vi "期末11 (1).vi"() -> ()   [LabVIEW 2014]
uses:
  <vilib>/vision/NI_Vision_Development_Module.lvlib
panel:
  in  "計數器":dbl
  out "座標和":dbl
  out "output array":dbl[](array[numeric])
  out "x/y":dbl
  out "Image Out 2":T1(plugin-control)
  out "ROI":T2
  in  "紀錄中點座標和":bool
  out "填入飽和磁場分量尖點座標和 2":dbl
  in  "3. Number of Erosion":i32=10
  out "Image Out":T1(plugin-control)
  in  "紀錄電流":dbl[](array[numeric])
  in  "Tab Control 2":enum32{"座標", "座標和", "作圖"}(tab)
  out "瞬間尖點座標":dbl[][](array[numeric])
  out "尖點座標和":dbl[](array[numeric])
  out "相減結果":dbl[](array[numeric])
  out "分量-電流":cluster{"紀錄電流":dbl[], dbl[]}(graph)
  in  "紀錄":bool
  in  "結束實驗":bool
  in  "1. 範圍選擇":T3={"色相（H）"={0, 255}, "飽和度（S）"={0, 255}, "亮度（L）"={0, 255}} {"亮度（L）" scale=0.0..255.0; "飽和度（S）" scale=0.0..255.0; "色相（H）" scale=0.0..255.0}
  out "Number of Particles":i32
  out "output cluster":cluster{"X":dbl, "Y":dbl}
  in  "Tab Control":T4(tab)
  out "1. 顏色選取":T1(plugin-control)
  out "2. 填補空隙":T1(plugin-control)
  out "3. 移除雜點":T1(plugin-control)
  out "4. 形狀修正":T1(plugin-control)
  out "5. 選取結果":T1(plugin-control)
  out "Particle Measurements":dbl[][](array[numeric])
  out "Error Out":errorcluster
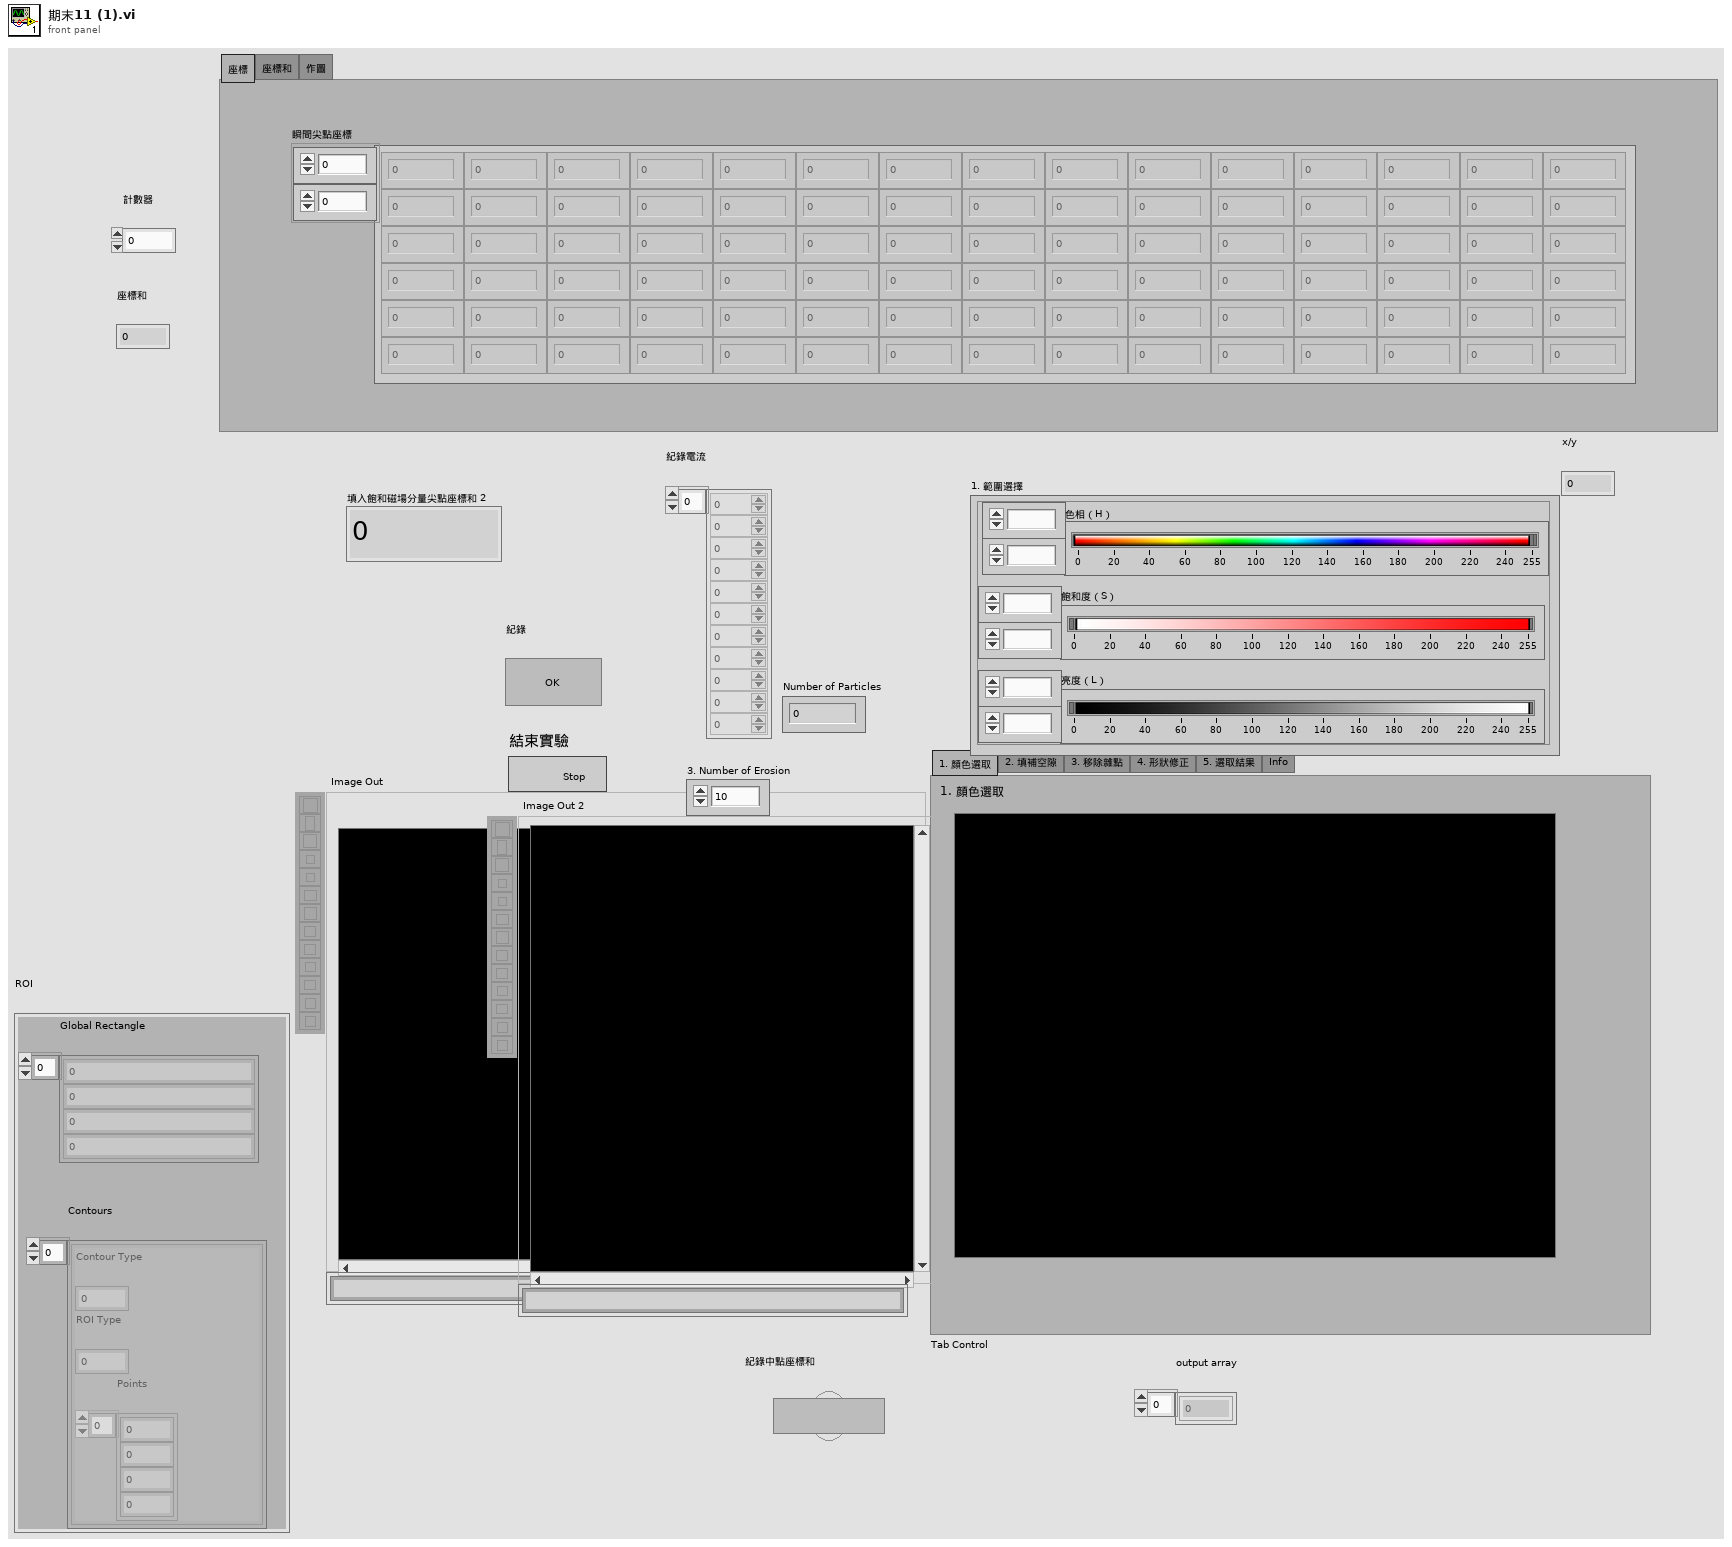
[diagram p1: front panel]
types:
  T1 = typedef "IMAQ Image.ctl" = refnum<image>
  T2 = cluster{"Global Rectangle":i32[], "Contours":cluster{"Contour Type":u32, "ROI Type":u32, "Points":i32[]}[]}
  T3 = cluster{"色相（H）":cluster{u8, u8}, "飽和度（S）":cluster{u8, u8}, "亮度（L）":cluster{u8, u8}}
  T4 = enum32{"1. 顏色選取", "2. 填補空隙", "3. 移除雜點", "4. 形狀修正", "5. 選取結果", "Info"}
  T5 = typedef "Image Type" = u32
  T6 = cluster{"Numeric":dbl, "Numeric":dbl, "Numeric":dbl, "Numeric":dbl}
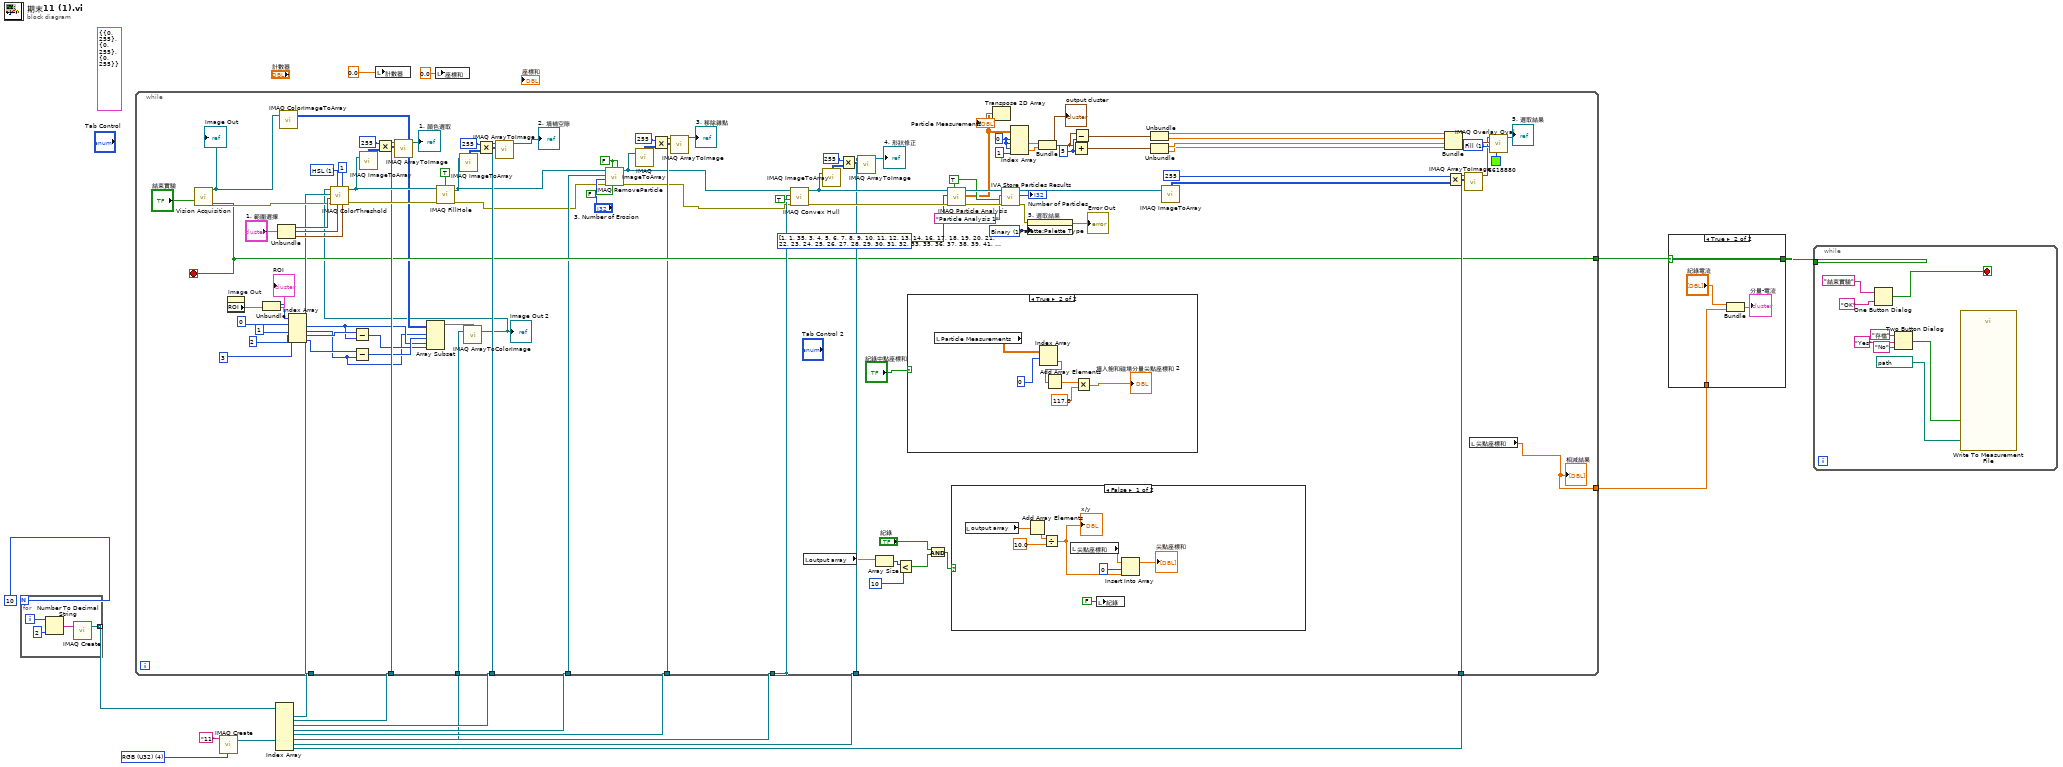
[diagram p0: block diagram]
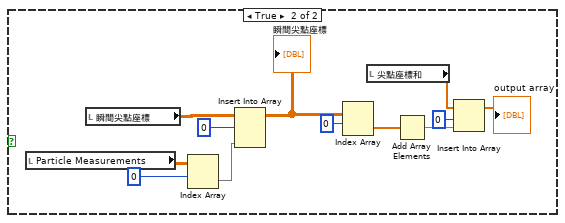
[diagram p3: hidden frame]
diagram:
  w5 = T5 4 items=["Grayscale (U8)", "Grayscale (I16)", "Grayscale (SGL)", "Complex (CSG)", "RGB (U32)", "HSL (U32)", "RGB (U64)", "Grayscale (U16)"] ("Image Type")
  (unwired) T3 {"色相（H）"={0, 255}, "飽和度（S）"={0, 255}, "亮度（L）"={0, 255}} ("範圍選擇")
  n1 = for {
    N: 10 -> [_]
    tunnel: [w19] -> w18 mode=indexing
    i -> [w21]
    n2 = Number To Decimal String(number=w21, width (-)=2) -> (decimal integer string=w20:string)
    n3 = call "IMAQ Create"("Image Name"=w20) -> ("New Image"=w19:T1)  [unwired: 4 in, 1 out]
  }
  n4 = call "IMAQ Create"("Image Name"="11", "Image Type"=w5) -> ("New Image"=w6:T1)  [unwired: 3 in, 1 out]
  n5 = Index Array(array=w18) -> (element #1=w17:T1, element #2=w16:T1, element #3=w15:T1, element #4=w8:T1, element #5=w7:T1, element #6=w13:T1, element #7=w12:T1, element #8=w11:T1)  [unwired: 8 in]
  n6 = while {
    tunnel: w15 -> [w95]
    tunnel: w13 -> [w106]
    tunnel: [w106] -> _
    tunnel: w16 -> [w100]
    tunnel: w17 -> [w94]
    tunnel: w12 -> [w88]
    tunnel: w11 -> [w65]
    tunnel: [w61] -> w10
    tunnel: [w47] -> w9
    tunnel: w8 -> [w54]
    tunnel: w7 -> [w53]
    tunnel: w6 -> [w37]
    stop <- w61 stop-if-true
    w58 = FALSE ("Connectivity 4/8 (8)")
    w70 = u32 1 items=["Frame", "Fill"] ("Drawing Mode (Frame)")
    w79 = 5
    w84 = 0
    w108 = u32 1 items=["Grayscale", "Binary", "Gradient", "Rainbow", "Temperature", "User Defined"] ("Palette")
    w113 = i32[] [1, 1, 35, 3, 4, 5, 6, 7, 8, 9, 10, 11, 12, 13, 14, 16, 17, 18, 19, 20, 21, 22, 23, 24, 25, 26, 27, 28, 29, 30, 31, 32, 33, 35, 36, 37, 38, 39, 41, 42, 43, 45, 46, 48, 49, 50, 51, 53, 54, 55, 56, 58, 59, 60, 61, 62, 63, 64, 65, 66, 68, 69, 70, 71, 72, 73, 74, 75, 76, 77, 78, 79, 80, 81, 82, 83, 84, 85, 86, 87, 88] items=["Center of Mass X", "Center of Mass Y", "First Pixel X", "First Pixel Y", "Bounding Rect Left", "Bounding Rect Top", "Bounding Rect Right", "Bounding Rect Bottom", "Max Feret Diameter Start X", "Max Feret Diameter Start Y", "Max Feret Diameter End X", "Max Feret Diameter End Y", "Max Horiz. Segment Length Left", "Max Horiz. Segment Length Right", "Max Horiz. Segment Length Row", "-", "Bounding Rect Width", "Bounding Rect Height", "Bounding Rect Diagonal", "Perimeter", "Convex Hull Perimeter", "Holes' Perimeter", "Max Feret Diameter", "Equivalent Ellipse Major Axis", "Equivalent Ellipse Minor Axis", "Equivalent Ellipse Minor Axis (Feret)", "Equivalent Rect Long Side", "Equivalent Rect Short Side", "Equivalent Rect Diagonal", "Equivalent Rect Short Side (Feret)", "Average Horiz. Segment Length", "Average Vert. Segment Length", "Hydraulic Radius", "Waddel Disk Diameter", "-", "Area", "Holes' Area", "Particle & Holes' Area", "Convex Hull Area", "Image Area", "-", "Number of Holes", "Number of Horiz. Segments", "Number of Vert. Segments", "-", "Orientation", "Max Feret Diameter Orientation", "-", "% Area/Image Area", "% Area/(Particle & Holes' Area)", "Ratio of Equivalent Ellipse Axes", "Ratio of Equivalent Rect Sides", "-", "Elongation Factor", "Compactness Factor", "Heywood Circularity Factor", "Type Factor", "-", "Sum X", "Sum Y", "Sum XX", "Sum XY", "Sum YY", "Sum XXX", "Sum XXY", "Sum XYY", "Sum YYY", "-", "Moment of Inertia XX", "Moment of Inertia XY", "Moment of Inertia YY", "Moment of Inertia XXX", "Moment of Inertia XXY", "Moment of Inertia XYY", "Moment of Inertia YYY", "Norm. Moment of Inertia XX", "Norm. Moment of Inertia XY", "Norm. Moment of Inertia YY", "Norm. Moment of Inertia XXX", "Norm. Moment of Inertia XXY", "Norm. Moment of Inertia XYY", "Norm. Moment of Inertia YYY", "Hu Moment 1", "Hu Moment 2", "Hu Moment 3", "Hu Moment 4", "Hu Moment 5", "Hu Moment 6", "Hu Moment 7"] ("Pixel Measurements")
    w115 = TRUE ("Connectivity 4/8 (8)")
    w124 = u16 1 items=["RGB", "HSL", "HSV", "HSI"] ("Color Mode")
    n7 = call "Vision Acquisition"("Stop (F)"="結束實驗") -> ("Image Out"=w45:T1, "Stopped"=w61:bool, "error out"=w119:errorcluster)  [unwired: 24 in]
    "Image Out" <- w45
    n8 = property on="Image Out" class="ImageControl"() -> ("ROI"=w43:T2)  [unwired: 2 in, 2 out]
    "ROI" <- w43
    n9 = Unbundle(w43) -> ("Global Rectangle"=w42:i32[])  [unwired: 1 out]
    n10 = Unbundle("1. 範圍選擇") -> ("色相（H）"=w123:cluster{u8, u8}, "飽和度（S）"=w122:cluster{u8, u8}, "亮度（L）"=w121:cluster{u8, u8})
    n11 = call "IMAQ ColorImageToArray"("Image"=w45) -> ("Image Pixels (U32)"=w44:u32[][])  [unwired: 3 in, 2 out]
    n12 = Index Array(array=w42, index #1=0 ("index"), index #2=1 ("index"), index #3=2 ("index"), index #4=3 ("index")) -> (element #1=w32:i32, element #2=w30:i32, element #3=w35:i32, element #4=w31:i32)
    n13 = Subtract(x=w35, y=w32) -> (x-y=w33:i32)
    n14 = Subtract(x=w31, y=w30) -> (x-y=w34:i32)
    n15 = Array Subset(array=w44, index (row)=w30, length (row)=w34, index (col)=w32, length (col)=w33) -> (w36:u32[][])
    n16 = call "IMAQ ArrayToColorImage"("Image Pixels (U32)"=w36, "Image"=w37) -> ("Image Out"=w29:T1)  [unwired: 3 in, 1 out]
    "Image Out 2" <- w29
    n17 = call "IMAQ ColorThreshold"("Blue or Luma or Val or Inten Range"=w121, "Replace Value"=1, "Green or Sat Range"=w122, "Color Mode"=w124, "error in (no error)"=w119, "Red or Hue Range"=w123, "Image Dst"=w94, "Image Src"=w29) -> ("error out"=w110:errorcluster, "Image Dst Out"=w105:T1)  [unwired: 2 out]
    n18 = call "IMAQ ImageToArray"("Image"=w105) -> ("Image Pixels (U8)"=w103:u8[][])  [unwired: 3 in, 4 out]
    n19 = Multiply(x=255, y=w103) -> (x*y=w102:i32[][])
    n20 = call "IMAQ ArrayToImage"("Image Pixels (U8)"=w102, "Image"=w100) -> ("Image Out"=→"1. 顏色選取":T1)  [unwired: 8 in, 1 out]
    n21 = call "IMAQ FillHole"("error in (no error)"=w110, "Image Src"=w105, "Connectivity 4/8 (8)"=TRUE) -> ("error out"=w52:errorcluster, "Image Dst Out"=w50:T1)  [unwired: 1 in, 2 out]
    n22 = call "IMAQ ImageToArray"("Image"=w50) -> ("Image Pixels (U8)"=w98:u8[][])  [unwired: 3 in, 4 out]
    n23 = Multiply(x=255, y=w98) -> (x*y=w99:i32[][])
    n24 = call "IMAQ ArrayToImage"("Image Pixels (U8)"=w99, "Image"=w95) -> ("Image Out"=→"2. 填補空隙":T1)  [unwired: 8 in, 1 out]
    n25 = call "IMAQ RemoveParticle"("Connectivity 4/8 (8)"=w58, "Low Pass/High Pass (Low)"=FALSE, "Square/Hexa (Square)"=w58, "error in (no error)"=w52, "Number of Erosion"="3. Number of Erosion", "Image Dst"=w54, "Image Src"=w50) -> ("error out"=w51:errorcluster, "Image Dst Out"=w49:T1)  [unwired: 3 out]
    n26 = call "IMAQ ImageToArray"("Image"=w49) -> ("Image Pixels (U8)"=w48:u8[][])  [unwired: 3 in, 4 out]
    n27 = Multiply(x=255, y=w48) -> (x*y=w56:i32[][])
    n28 = call "IMAQ ArrayToImage"("Image Pixels (U8)"=w56, "Image"=w53) -> ("Image Out"=→"3. 移除雜點":T1)  [unwired: 8 in, 1 out]
    n29 = call "IMAQ Convex Hull"("error in (no error)"=w51, "Connectivity 4/8 (8)"=TRUE, "Image Dst"=w106, "Image Src"=w49) -> ("error out"=w114:errorcluster, "Image Dst Out"=w89:T1)  [unwired: 6 out]
    n30 = local read "output array"() -> (w23:dbl[])
    n31 = call "IMAQ ImageToArray"("Image"=w89) -> ("Image Pixels (U8)"=w92:u8[][])  [unwired: 3 in, 4 out]
    n32 = Multiply(x=255, y=w92) -> (x*y=w93:i32[][])
    n33 = call "IMAQ ArrayToImage"("Image Pixels (U8)"=w93, "Image"=w88) -> ("Image Out"=→"4. 形狀修正":T1)  [unwired: 8 in, 1 out]
    n34 = Array Size(array=w23) -> (size(s)=w27:i32)
    n35 = Less?(x=w27, y=10) -> (x < y?=w25:bool)
    n36 = case shown="True" "紀錄中點座標和" {
      frame False {
      }
      frame True {
        n37 = local read "Particle Measurements"() -> (w150:dbl[][])
        n38 = Index Array(array=w150, index (row)=0) -> (element=w149:dbl[])  [unwired: 1 in]
        n39 = Add Array Elements(numeric array=w149) -> (sum=w148:dbl)
        n40 = Multiply(x=w148, y=117.0) -> (x*y=→"填入飽和磁場分量尖點座標和 2":dbl)
      }
    }
    n41 = And(x="紀錄", y=w25) -> (x .and. y?=w24:bool)
    n42 = call "IMAQ Particle Analysis"("Connectivity 4/8 (8)"=w115, "error in (no error)"=w114, "Pixel Measurements"=w113, "Image"=w89) -> ("error out"=w118:errorcluster, "Particle Measurements (Pixels)"=w85:dbl[][], "Image Out (duplicate)"=w116:T1)  [unwired: 1 in, 4 out]
    n43 = case shown="False" w24 {
      frame False {
        n44 = local read "output array"() -> (w131:dbl[])
        n45 = Add Array Elements(numeric array=w131) -> (sum=w132:dbl)
        n46 = Divide(x=w132, y=10.0) -> (x/y=w128:dbl)
        "x/y" <- w128
        n47 = local read "尖點座標和"() -> (w130:dbl[])
        n48 = local write "紀錄"(FALSE ("紀錄")) -> ()
        n49 = Insert Into Array(array=w130, index=0, new element=w128) -> (→"尖點座標和":dbl[])
      }
      frame True {
        n50 = local read "Particle Measurements"() -> (w136:dbl[][])
        n51 = local read "瞬間尖點座標"() -> (w141:dbl[][])
        n52 = Index Array(array=w136, index (row)=0) -> (element=w140:dbl[])  [unwired: 1 in]
        n53 = Insert Into Array(array=w141, index (row)=0 ("index"), new element=w140) -> (w143:dbl[][])  [unwired: 1 in]
        "瞬間尖點座標" <- w143
        n54 = Index Array(array=w143, index (row)=0) -> (element=w145:dbl[])  [unwired: 1 in]
        n55 = local read "尖點座標和"() -> (w137:dbl[])
        n56 = Add Array Elements(numeric array=w145) -> (sum=w139:dbl)
        n57 = Insert Into Array(array=w137, index=0 ("index (row)"), new element=w139) -> (→"output array":dbl[])
      }
    }
    n58 = Transpose 2D Array(2D array=w85) -> (transposed array=→"Particle Measurements":dbl[][])
    n59 = call <vilib>:"IVA Store Particles Results.vi"("error in (no error)"=w118, "Connectivity 4/8 (8)"=w115, "Step Name"="Particle Analysis 1", "Image in"=w116) -> ("error out"=w109:errorcluster, "Number of Particles"=→"Number of Particles":i32, "Image dup"=w69:T1)  [unwired: 5 out]
    n60 = Index Array(array=w85, index (row) #1=w84, index (col) #1=w84, index (row) #2=w84, index (col) #2=1) -> (element #1=w82:dbl, element #2=w81:dbl)
    n61 = property on="5. 選取結果" class="ImageControl"(error in=w109, "Palette:Palette Type"=w108) -> (error out=→"Error Out":errorcluster)  [unwired: 1 in, 1 out]
    n62 = Bundle("Numeric"=w82, "Numeric"=w81) -> (w78:cluster{"Numeric":dbl, "Numeric":dbl})  [unwired: 1 in]
    "output cluster" <- w78
    n63 = Add(x=w78, y=w79) -> (x+y=w76:cluster{"Numeric":dbl, "Numeric":dbl})
    n64 = Subtract(x=w78, y=w79) -> (x-y=w77:cluster{"Numeric":dbl, "Numeric":dbl})
    n65 = Unbundle(w77) -> ("Numeric"=w75:dbl, "Numeric"=w74:dbl)
    n66 = Unbundle(w76) -> ("Numeric"=w73:dbl, "Numeric"=w72:dbl)
    n67 = call "IMAQ ImageToArray"("Image"=w69) -> ("Image Pixels (U8)"=w66:u8[][])  [unwired: 3 in, 4 out]
    n68 = Bundle("Numeric"=w75, "Numeric"=w74, "Numeric"=w73, "Numeric"=w72) -> (w71:T6)  [unwired: 1 in]
    n69 = Multiply(x=255, y=w66) -> (x*y=w67:i32[][])
    n70 = call "IMAQ ArrayToImage"("Image Pixels (U8)"=w67, "Image"=w65) -> ("Image Out"=w64:T1)  [unwired: 8 in, 1 out]
    n71 = local read "尖點座標和"() -> (w47:dbl[])
    "相減結果" <- w47
    n72 = call "IMAQ Overlay Oval"("Color"=u32 6618880, "Drawing Mode (Frame)"=w70, "Bounding Rectangle"=w71, "Image"=w64) -> ("Image Out"=→"5. 選取結果":T1)  [unwired: 6 in, 1 out]
  }
  n73 = local write "計數器"(0.0 ("計數器")) -> ()
  n74 = local write "座標和"(0.0 ("座標和")) -> ()
  n75 = case shown="True" w10 {
    selector: w10 -> [w152 w156]
    tunnel: [w152 w156] -> w3
    tunnel: w9 -> [_ w155]
    frame False {
    }
    frame True {
      n76 = Bundle("紀錄電流"="紀錄電流", "尖點座標和"=w155) -> (→"分量-電流":cluster{"紀錄電流":dbl[], "尖點座標和":dbl[]})  [unwired: 1 in]
    }
  }
  n77 = while {
    tunnel: w3 -> [_]
    stop <- w164 stop-if-true
    n78 = One Button Dialog(message="結束實驗", button name ("OK")="OK") -> (true=w164:bool)
    n79 = Two Button Dialog(message="存檔", 1:"No" ("F button name (\"Cancel\")"), 2:"Yes" ("T button name (\"OK\")")) -> (T button?=w158:bool)
    n80 = call "Write To Measurement File"("Enable"=w158, "Filename"=path "實驗數據") -> ()  [unwired: 15 in, 3 out]
  }
